vi "TEST - MD5 Message Digest - Hexadecimal String.vi"(8 "error in (no error)":errorcluster) -> (0 "error out":errorcluster, 2 "Pass":bool)   [LabVIEW 2009]
uses:
  source/library/MD5 Message Digest/MD5 Message Digest (Hexadecimal String).vi
panel:
  out "Failures":T1(array[cluster])
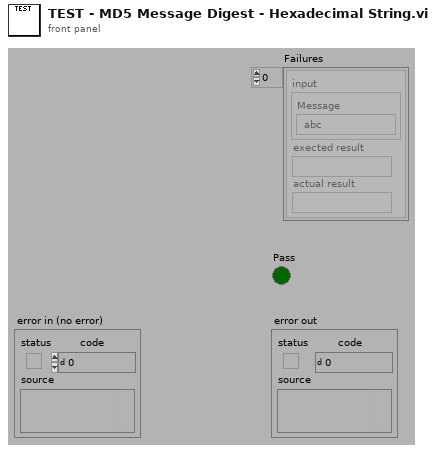
[diagram p1: front panel]
types:
  T1 = cluster{"input":cluster{"Message":string}, "exected result":string, "actual result":string}[]
  T2 = cluster{"input":cluster{"Message":string}, "exected result":string, "actual result":string}
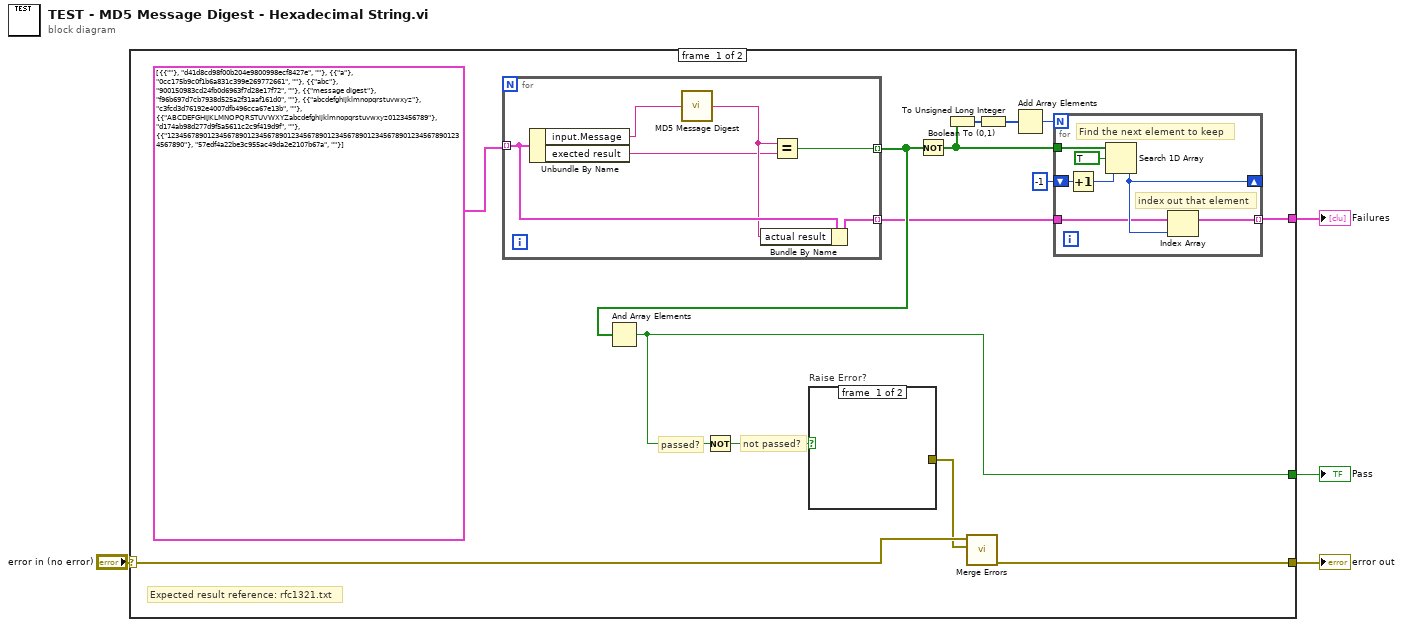
[diagram p0: block diagram]
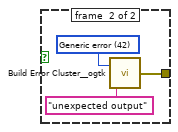
[diagram p2: hidden frame]
diagram:
  n1 = case shown="No Error" "error in (no error)" {
    selector: "error in (no error)" -> [w18 w35]
    tunnel: [w14 _] -> w4
    tunnel: [w17 w35] -> w2
    tunnel: [w6 _] -> w1
    frame #0 {
      # "Expected result reference: rfc1321.txt"
      # "not passed?"
      # "passed?"
      n2 = for {
        tunnel: T1 [{"input"={"Message"=""}, "exected result"="d41d8cd98f00b204e9800998ecf8427e", "actual result"=""}, {"input"={"Message"="a"}, "exected result"="0cc175b9c0f1b6a831c399e269772661", "actual result"=""}, {"input"={"Message"="abc"}, "exected result"="900150983cd24fb0d6963f7d28e17f72", "actual result"=""}, {"input"={"Message"="message digest"}, "exected result"="f96b697d7cb7938d525a2f31aaf161d0", "actual result"=""}, {"input"={"Message"="abcdefghijklmnopqrstuvwxyz"}, "exected result"="c3fcd3d76192e4007dfb496cca67e13b", "actual result"=""}, {"input"={"Message"="ABCDEFGHIJKLMNOPQRSTUVWXYZabcdefghijklmnopqrstuvwxyz0123456789"}, "exected result"="d174ab98d277d9f5a5611c2c9f419d9f", "actual result"=""}, {"input"={"Message"="12345678901234567890123456789012345678901234567890123456789012345678901234567890"}, "exected result"="57edf4a22be3c955ac49da2e2107b67a", "actual result"=""}] -> [w29] mode=indexing
        tunnel: [w31] -> w8 mode=indexing
        tunnel: [w30] -> w7 mode=indexing
        n3 = Unbundle By Name(w29) -> ("input.Message"=w28:string, "exected result"=w26:string)
        n4 = call-poly "MD5 Message Digest.vi"("Message"=w28) -> ("MD5 Message Digest"=w27:string)
        n5 = Bundle By Name(cluster=w29, "actual result"=w27) -> (w30:T2)
        n6 = Equal?(x=w27, y=w26) -> (x = y?=w31:bool)
      }
      n7 = And Array Elements(Boolean array=w8) -> (logical AND=w14:bool)
      n8 = Not(x=w14) -> (.not. x?=w15:bool)
      n9 = case "Raise Error?" shown="True" w15 {
        tunnel: [_ w32] -> w16
        frame #0 {
        }
        frame #1 {
          w33 = 42 items=["No error", "Argument error", "Memory is full", "Out of zone", "End of file", "File already open", "Generic file I/O error", "File not found", "File permission error", "Disk is full", "Duplicate path", "Too many files open", "System feature not enabled", "Resource file not found", "Cannot add resource", "Resource not found", "Image not found", "Image memory error", "Pen does not exist", "Config type invalid", "Config token not found", "Config parse error", "Config memory error", "Bad external code format", "Bad external code offset", "External code not present", "Null window", "Destroy window error", "Null menu", "Print aborted", "Bad print record", "Print driver error", "Windows error during printing", "Memory error during printing", "Print dialog error", "Generic print error", "Invalid device refnum", "Device not found", "Device parameter error", "Device unit error", "Cannot open device", "Device call aborted", "Generic error", "Cancelled by user", "Object ID too low", "Object ID too high", "Object not in heap", "Unknown heap", "Unknown object (invalid DefProc)", "Unknown object (DefProc not in table)", "Message out of range", "Invalid (null) method", "Unknown message", "Manager call not supported", "Bad address", "Network operation in progress", "Network operation timed out", "Connection is busy", "Network attribute not supported", "Network error", "Address in use", "System out of memory", "Connection aborted", "Connection refused", "Not connected", "Already connected", "Connection closed", "Initialization error (interapplication manager)", "Bad occurrence", "Wait on unbound occurrence handler", "Occurrence queue overflow", "Datalog type conflict", "Unused", "Unrecognized type (interapplication manager)", "Memory corrupt", "Failed to make temporary DLL", "Old CIN version", "Drag socket not found", "Failed to load drop-object", "Failed to register OLE object", "Failed to release OLE object", "Format specifier type mismatch", "Unknown format specifier", "Too few format specifiers", "Too many format specifiers", "Scan failed", "Newer CIN version", "Error converting to variant", "Runtime menu error", "Password tampered", "Variant attribute not found", "Incompatible variant data type", "Event data is not available", "Event Store is not present", "Occurrence is not found", "Event Queue is not created", "Event info is not available", "Refnum passed is NULL", "Error retrieving Class GUID", "Error retrieving CoClass GUID", "Error retrieving TypeLib GUID.", "Bad built application magic bytes.", "Specific driver is different from the specific driver associated with the Logical Name.", "There is no session opened to the class driver.", "Max Error", "MAX - Error with config objects", "MAX - Error loading configuration", "MAX - Group not supported"]
          n10 = call <userlib>:"Build Error Cluster__ogtk.vi"("String to Prepend to source (\"\")"="unexpected output" ("String to Prepend to source (\"\")"), "code"=w33) -> ("error out"=w32:errorcluster)
        }
      }
      n11 = Not(x=w8) -> (.not. x?=w10:bool[])
      n12 = Boolean To (0,1)(Boolean=w10) -> (0, 1=w11:i16[])
      n13 = call <vilib>:"Merge Errors.vi"("error in 2 (no error)"=w16, "error in 1 (no error)"=w18) -> ("error out"=w17:errorcluster)  [unwired: 5 in]
      n14 = To Unsigned Long Integer(number=w11) -> (unsigned 32bit integer=w9:u32[])
      n15 = Add Array Elements(numeric array=w9) -> (sum=w12:u32)
      n16 = for {
        N: w12 -> [_]
        tunnel: w7 -> [w21]
        tunnel: w10 -> [w25]
        shift-right: [w22] -> _
        shift-left: -1 ("start index (0)") -> [w23]
        tunnel: [w20] -> w6 mode=indexing
        # "index out that element"
        # "Find the next element to keep"
        n17 = Increment(x=w23) -> (x+1=w19:i32)
        n18 = Search 1D Array(1D array=w25, element=TRUE, start index (0)=w19) -> (index of element=w22:i32)
        n19 = Index Array(array=w21, index=w22) -> (element=w20:T2)
      }
    }
    frame #1 {
    }
  }
  "Pass" <- w4
  "error out" <- w2
  "Failures" <- w1
